vi "Hide VI Panel.vi"(8 "error in":errorcluster, 11 "VI":refnum<vi>) -> (0 "error out":errorcluster)   [LabVIEW 2026, in "Settings Editor.lvlib"]
doc: "Hide the panel of the specified VI.\n_____\nBased on DQMH Project Template 4.0.0.47.\n_____\nBased on DQMH Dev Tools: Project Template 7.1.2.1547."
uses:
  Settings Editor.lvlib
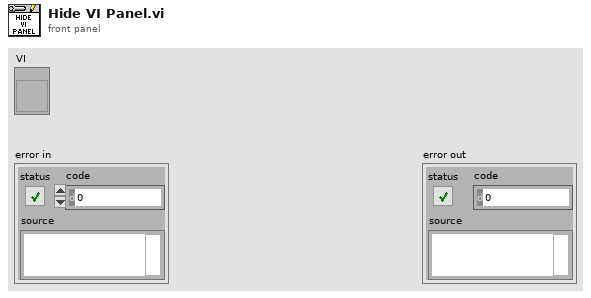
[diagram p1: front panel]
types:
  T1 = enum32{"Invalid", "Standard", "Closed", "Hidden", "Minimized", "Maximized"}
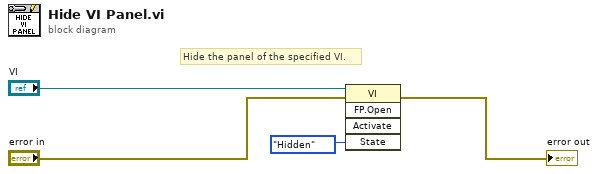
[diagram p0: block diagram]
diagram:
  # "Hide the panel of the specified VI."
  n1 = invoke on="Invoke Node" class="VI" method="FP.Open"(reference="VI", error in="error in", "State"=T1."Hidden") -> (error out=→"error out":errorcluster)  [unwired: 2 in, 4 out]
